vi "Diag_90.vi"(0 "GEA2 Reference In":refnum<k24>, 5 "GEA Inputs":T1={"Source"=228, "Destination"=0} {"Destination" format="%.0x"; "Source" format="%.0x"}, 11 "Error In":errorcluster) -> (4 "GEA2 Reference Out":refnum<k24>, 6 "Diagnostics Entity Count":u8, 8 "Diagnostic Entity Map Location":u16 format="%.0x", 15 "Error Out":errorcluster)   [LabVIEW 2023]
uses:
  D:/Common/LabVIEW GEA2 Toolkit/source/GEA3 DLL Source/GeaCommunication.dll
  LabVIEW GEA2 Toolkit/source/GEA3 DLL Source/GeaCommunication.dll
  LabVIEW GEA2 Toolkit/GEA3/type defs/Source_Destination.ctl
  LabVIEW GEA2 Toolkit/GEA3/type defs/ERD Read Data In.ctl
  LabVIEW GEA2 Toolkit/GEA3/library/GEA2_Toolkit.lvlib
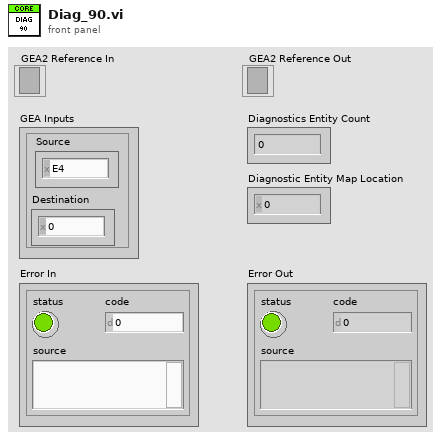
[diagram p1: front panel]
types:
  T1 = typedef "Source_Destination.ctl" = cluster{"Source":u8, "Destination":u8}
  T2 = typedef "ERD Read Data In.ctl" = cluster{"ERD Number":u16, "Data Type":enum16{"string", "boolean", "uint8_t", "uint16_t", "uint32_t", "uint64_t", "int8_t", "int16_t", "int32_t", "int64_t"}}
  T3 = typedef "ERD Read Data Out.ctl" = cluster{"ERD Number":u16, "Data":string}
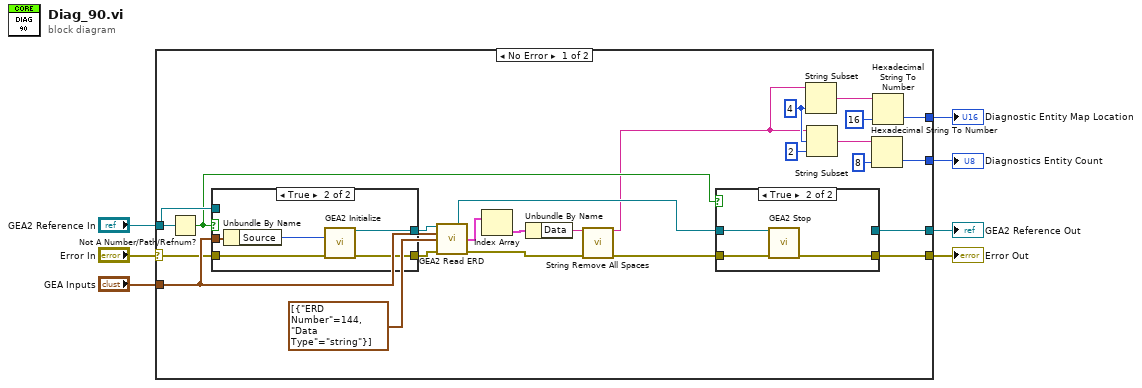
[diagram p0: block diagram]
diagram:
  n1 = case shown="No Error" "Error In" {
    selector: "Error In" -> [w18 w45]
    tunnel: [w17 w45] -> w7
    tunnel: "GEA2 Reference In" -> [w31 w44]
    tunnel: "GEA Inputs" -> [w24 _]
    tunnel: [w19 w44] -> w4
    tunnel: [w8 _] -> w1
    tunnel: [w9 _] -> w2
    frame No Error {
      w11 = 4 ("length (rest)")
      n2 = Not A Number/Path/Refnum?(number/path/refnum=w31) -> (NaN/Path/Refnum?=w20:bool)
      n3 = case shown="True" w20 {
        tunnel: w18 -> [w37 w43]
        tunnel: w24 -> [_ w42]
        tunnel: [w37 w41] -> w29
        tunnel: [w38 w40] -> w28
        tunnel: w31 -> [w38 _]
        frame False {
        }
        frame True {
          n4 = Unbundle By Name(w42) -> ("Source"=w39:u8)
          n5 = call "GEA2 Initialize.vi"("Source Address"=w39, "error in"=w43) -> ("GEA2 Reference Out"=w40:refnum<k24>, "error out"=w41:errorcluster)  [unwired: 10 in, 2 out]
        }
      }
      n6 = call "GEA2 Read ERD.vi"("GEA2 Reference In"=w28, "GEA Inputs"=w24, "Read ERD List"=T2[] [{"ERD Number"=144, "Data Type"=enum."string"}], "Error In"=w29) -> ("GEA2 Reference Out"=w21:refnum<k24>, "ERD Data Out"=w26:T3[], "Error Out"=w27:errorcluster)  [unwired: 8 in, 1 out]
      n7 = Index Array(array=w26) -> (element=w25:T3)  [unwired: 1 in]
      n8 = Unbundle By Name(w25) -> ("Data"=w30:string)
      n9 = call "String Remove All Spaces.vi"("Input String"=w30, "error in (no error)"=w27) -> ("Spaces Removed"=w10:string, "error out"=w22:errorcluster)  [unwired: 12 in]
      n10 = case shown="True" w20 {
        tunnel: w22 -> [w32 w36]
        tunnel: [w32 w35] -> w17
        tunnel: [w33 _] -> w19
        tunnel: w21 -> [w33 w34]
        frame False {
        }
        frame True {
          n11 = call "GEA2 Stop.vi"("GEA2 Reference In"=w34, "Error In"=w36) -> ("Error Out"=w35:errorcluster)  [unwired: 13 in]
        }
      }
      n12 = String Subset(string=w10, length (rest)=w11) -> (substring=w13:string)  [unwired: 1 in]
      n13 = String Subset(string=w10, offset (0)=w11, length (rest)=2 ("length (rest)")) -> (substring=w14:string)
      n14 = Hexadecimal String To Number(string=w14, default (0uL)=u8 8 ("default (0 U32)")) -> (number=w8:u8)  [unwired: 1 in, 1 out]
      n15 = Hexadecimal String To Number(string=w13, default (0uL)=u16 16 ("default (0 U32)")) -> (number=w9:u16)  [unwired: 1 in, 1 out]
    }
    frame Error {
    }
  }
  "Error Out" <- w7
  "GEA2 Reference Out" <- w4
  "Diagnostic Entity Map Location" <- w2
  "Diagnostics Entity Count" <- w1
